vi "Test Empty Dictionary.vi"(8 "error in (no error)":errorcluster) -> (0 "error out":errorcluster)   [LabVIEW 2020]
doc: "Test case to validate the dictionary is empty."
uses:
  Classes/Integer Dictionary.lvclass
  classes/Assert/Assert.lvclass
  classes/Test/Test.lvclass
panel:
  # "See block diagram"
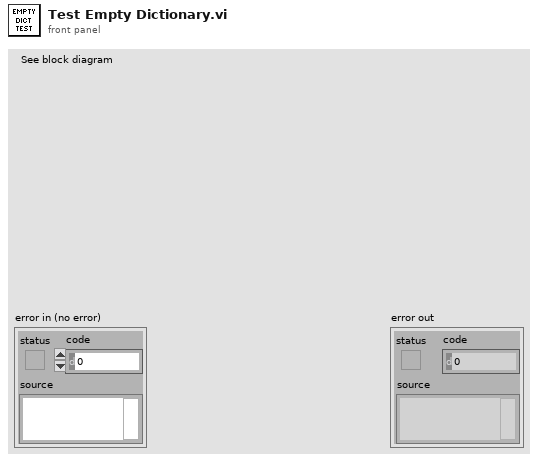
[diagram p1: front panel]
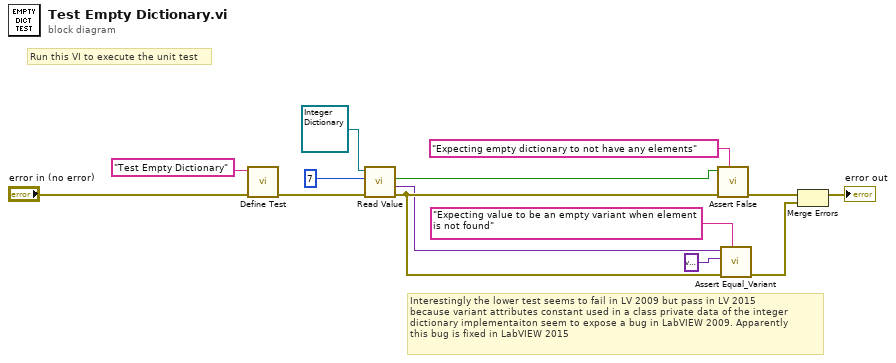
[diagram p0: block diagram]
diagram:
  # "Run this VI to execute the unit test"
  # "Interestingly the lower test seems to fail in LV 2009 but pass in LV 2015\nbecause variant attributes constant used in a class private data of the integer \ndictionary implementaiton seem to expose a bug in LabVIEW 2009. Apparently\nthis bug is fixed in LabVIEW 2015"
  n1 = call "Define Test.vi"("error in (no error)"="error in (no error)", "Label (VI Title)"="Test Empty Dictionary") -> ("error out"=w6:errorcluster)  [unwired: 8 in, 1 out]
  n2 = call "Read Value.vi"("error in (no error)"=w6, "Key"=7, "Integer Dictionary in"=refnum<class "Integer Dictionary.lvclass"> refnum ("Integer Dictionary.lvclass")) -> ("error out"=w11:errorcluster, "Value"=w10:variant, "found?"=w13:bool)  [unwired: 5 in, 1 out]
  n3 = call "Assert False.vi"("Label"="Expecting empty dictionary to not have any elements", "error in (no error)"=w11, "False?"=w13) -> ("error out"=w3:errorcluster)  [unwired: 7 in, 1 out]
  n4 = call "Assert Equal_Variant.vi"("Label"="Expecting value to be an empty variant when element is not found", "error in (no error)"=w11, "Y"=variant, "X"=w10) -> ("error out"=w2:errorcluster)  [unwired: 7 in]
  n5 = Merge Errors(w3, w2) -> (→"error out":errorcluster)
